vi "搬运盲元表到DDR.vi"(8 "error in":errorcluster) -> (0 "error out":errorcluster, 2 "return":i32)   [LabVIEW 2016]
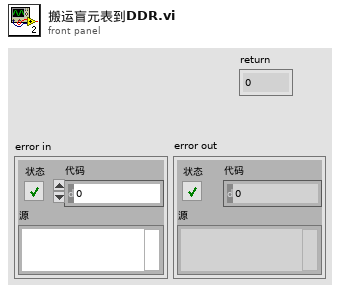
[diagram p1: front panel]
types:
  T1 = cluster{"byCmdType":u8, "bySubCmd":u8, "byParam_h":u8, "byParam_l":u8, "byAddr1_hh":u8, "byAddr1_h":u8, "byAddr1_l":u8, "byAddr1_ll":u8, "byAddr2_hh":u8, "byAddr2_h":u8, "byAddr2_l":u8, "byAddr2_ll":u8, "byLen_hh":u8, "byLen_h":u8, "byLen_l":u8, "byLen_ll":u8}
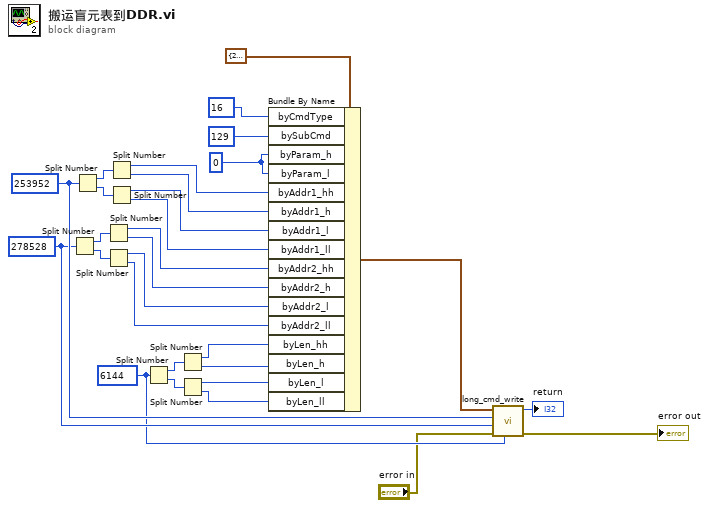
[diagram p0: block diagram]
diagram:
  w4 = 6144
  w19 = u8 0 ("byParam_h")
  w20 = 278528
  w21 = 253952
  n1 = Split Number(x=w20) -> (hi(x)=w23:u16, lo(x)=w24:u16)
  n2 = Split Number(x=w21) -> (hi(x)=w26:u16, lo(x)=w25:u16)
  n3 = Split Number(x=w23) -> (hi(x)=w14:u8, lo(x)=w13:u8)
  n4 = Split Number(x=w24) -> (hi(x)=w12:u8, lo(x)=w11:u8)
  n5 = Split Number(x=w26) -> (hi(x)=w18:u8, lo(x)=w17:u8)
  n6 = Split Number(x=w25) -> (hi(x)=w16:u8, lo(x)=w15:u8)
  n7 = Split Number(x=w4) -> (hi(x)=w10:u16, lo(x)=w9:u16)
  n8 = Split Number(x=w10) -> (hi(x)=w8:u8, lo(x)=w7:u8)
  n9 = Split Number(x=w9) -> (hi(x)=w6:u8, lo(x)=w5:u8)
  n10 = Bundle By Name(cluster=T1 {"byCmdType"=24, "bySubCmd"=129, "byParam_h"=0, "byParam_l"=0, "byAddr1_hh"=0, "byAddr1_h"=0, "byAddr1_l"=0, "byAddr1_ll"=0, "byAddr2_hh"=0, "byAddr2_h"=0, "byAddr2_l"=0, "byAddr2_ll"=0, "byLen_hh"=0, "byLen_h"=0, "byLen_l"=0, "byLen_ll"=0} ("vd_cmd_long_header_t"), "byCmdType"=16, "bySubCmd"=129, "byParam_h"=w19, "byParam_l"=w19, "byAddr1_hh"=w18, "byAddr1_h"=w17, "byAddr1_l"=w16, "byAddr1_ll"=w15, "byAddr2_hh"=w14, "byAddr2_h"=w13, "byAddr2_l"=w12, "byAddr2_ll"=w11, "byLen_hh"=w8, "byLen_h"=w7, "byLen_l"=w6, "byLen_ll"=w5) -> (w22:T1)
  n11 = call "long_cmd_write.vi"("dwLen"=w4, "error in"="error in", "dwAddr2"=w20, "dwAddr1"=w21, "vd_cmd_long_header_t"=w22) -> ("error out"=→"error out":errorcluster, "return"=→"return":i32)  [unwired: 5 in]
